vi "Invert u8.vi"(11 "In (u8)":u8) -> (3 "Out (u8)":u8)   [LabVIEW 2015]
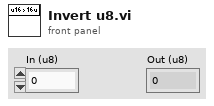
[diagram p1: front panel]
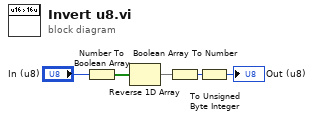
[diagram p0: block diagram]
diagram:
  n1 = Number To Boolean Array(number="In (u8)") -> (Boolean array=w5:bool[])
  n2 = Reverse 1D Array(array=w5) -> (reversed array=w4:bool[])
  n3 = Boolean Array To Number(Boolean array=w4) -> (number=w3:u32)
  n4 = To Unsigned Byte Integer(number=w3) -> (unsigned 8bit integer=→"Out (u8)":u8)
